vi "VIG - Ring Image Repository.vi"(7 "Method (Read)":enum16{"Read Data", "Write Data"}(ring), 8 "error in (no error)":errorcluster, 11 "Variant Data In":variant) -> (0 "error out":errorcluster, 3 "Variant Data Out":variant)   [LabVIEW 2017, in "Front Panel Publisher.lvlib" / "Select.lvclass"]
doc: "This is an example VIG or Functional global that can be used as a template. Replace the Variant Data In, and Variant Data Out with the data type you want, or use a Variant Repository."
uses:
  Select.lvclass
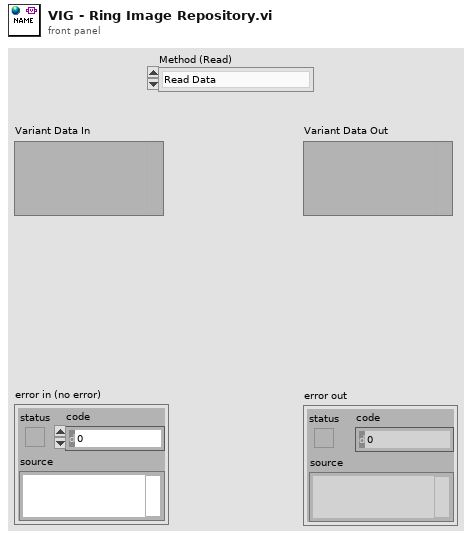
[diagram p1: front panel]
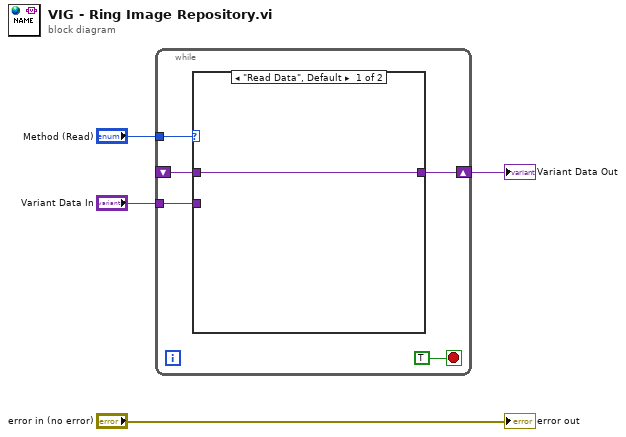
[diagram p0: block diagram]
diagram:
  n1 = while {
    tunnel: "Method (Read)" -> [w9]
    tunnel: "Variant Data In" -> [w8]
    shift-right: [w7] -> w1
    shift-left: _ -> [w6]
    stop <- TRUE stop-if-true
    n2 = case shown="\"Read Data\", Default" w9 {
      tunnel: w8 -> [_ w11]
      tunnel: [w10 w11] -> w7
      tunnel: w6 -> [w10 _]
      frame "Read Data", Default {
      }
      frame "Write Data" {
      }
    }
  }
  "Variant Data Out" <- w1
  "error out" <- "error in (no error)"
